vi "TPZ001.vi"() -> ()   [LabVIEW 2015]
panel:
  in  "ActiveX Container":refnum<k7>(container)
  out "X Position":sgl
  out "error out":errorcluster
  in  "APTPZMotor":refnum<k7>(container)
  in  "Serial":i32=81865521
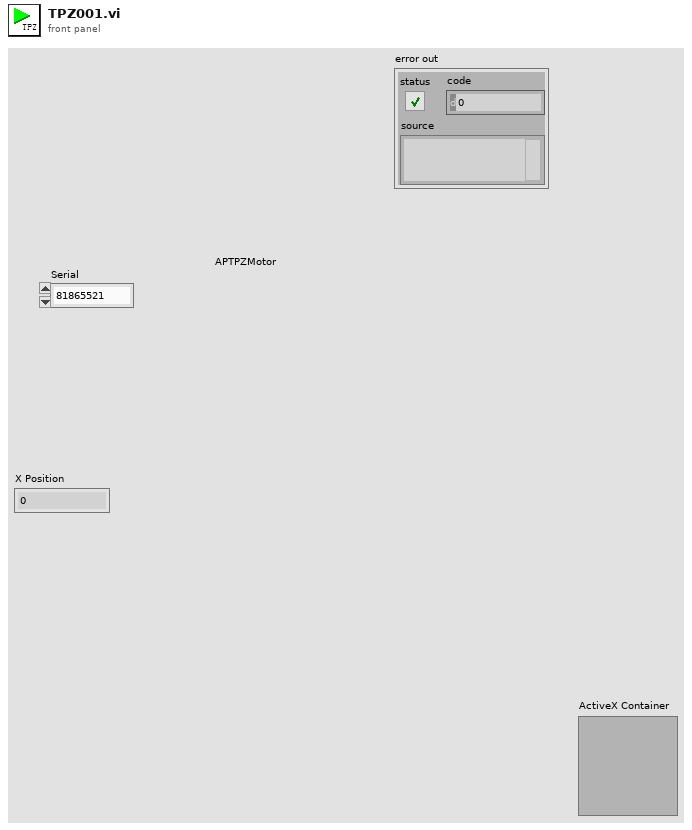
[diagram p1: front panel]
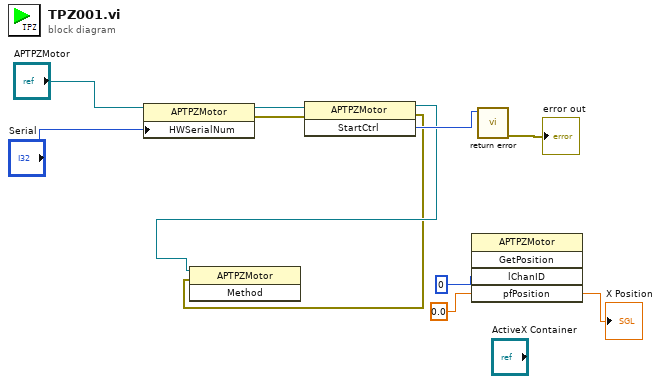
[diagram p0: block diagram]
diagram:
  n1 = property class="APTPZMotor"(reference="APTPZMotor", "HWSerialNum"="Serial") -> (reference out=w9:refnum<k7>, error out=w8:errorcluster)  [unwired: 1 in]
  n2 = invoke class="APTPZMotor" method="StartCtrl"(reference=w9, error in=w8) -> (reference out=w2:refnum<k7>, error out=w1:errorcluster, "StartCtrl"=w7:i32)  [unwired: 1 in]
  n3 = invoke class="APTPZMotor" method=#-1(reference=w2, error in=w1) -> ()  [unwired: 1 in, 3 out]
  n4 = invoke class="APTPZMotor" method="GetPosition"("lChanID"=0, "pfPosition"=sgl 0.0) -> ("pfPosition"=→"X Position":sgl)  [unwired: 3 in, 4 out]
  n5 = call "return error.vi"("return code"=w7) -> ("error out"=→"error out":errorcluster)  [unwired: 10 in]
